vi "MENU7.vi"   [LabVIEW 2015, in "Lazyboots Menu Tool Launch.lvlib"]
uses:
  _Library/Lazyboots Menu Tool Launch.lvlib
  <vilib>/Utility/config.llb/Read Key (String).vi
  <vilib>/Utility/config.llb/NI_LVConfig.lvlib
panel:
  # "Launching..."
types:
  T1 = enum32{"Invalid", "Standard", "Closed", "Hidden", "Minimized", "Maximized"}
  T2 = typedef "NI_LVConfig.lvlib/Config Data RefNum.ctl" = refnum<k1>
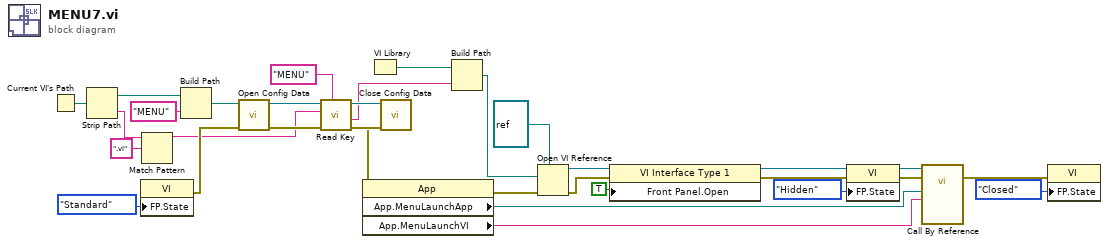
[diagram p0: block diagram]
diagram:
  n1 = Current VI's Path() -> (path=w30:path)
  n2 = Strip Path(path=w30) -> (stripped path=w29:path, name=w19:string)
  n3 = property class="VI"("FP.State"=T1."Standard" ("Front Panel Window:State")) -> (error out=w21:errorcluster)  [unwired: 2 in, 1 out]
  n4 = Match Pattern(string=w19, regular expression=".vi") -> (before substring=w18:string)  [unwired: 4 out]
  n5 = Build Path(base path=w29, name or relative path="MENU") -> (appended path=w27:path)
  n6 = call <vilib>:"Open Config Data.vi"("error in (no error)"=w21, "configuration file path"=w27) -> ("error out"=w25:errorcluster, "refnum"=w26:T2)  [unwired: 7 in, 1 out]
  n7 = call-poly <vilib>:"Read Key.vi"("section"="MENU", "error in (no error)"=w25, "key"=w18, "refnum"=w26) -> ("error out"=w22:errorcluster, "value"=w15:string, "refnum out"=w23:T2)  [unwired: 2 in, 3 out]
  n8 = VI Library() -> (path=w1:path)
  n9 = call <vilib>:"Close Config Data.vi"("error in (no error)"=w22, "refnum"=w23) -> ("error out"=w20:errorcluster)  [unwired: 1 in, 8 out]
  n10 = property class="App"(error in=w20) -> (error out=w14:errorcluster, "App.MenuLaunchApp"=w10:refnum<vi>, "App.MenuLaunchVI"=w9:string)  [unwired: 1 in, 1 out]
  n11 = Build Path(base path=w1, name or relative path=w15) -> (appended path=w16:path)
  n12 = Open VI Reference(type specifier VI Refnum (for type only)=refnum<vi> refnum, vi path=w16, error in (no error)=w14) -> (vi reference=w11:refnum<vi>, error out=w3:errorcluster)  [unwired: 3 out]
  n13 = property class="VI Interface Type 1"(reference=w11, error in=w3, "Front Panel.Open"=TRUE ("Front Panel Window:Open")) -> (reference out=w7:refnum<vi>, error out=w2:errorcluster)
  n14 = property class="VI"(error in=w2, "FP.State"=T1."Hidden" ("Front Panel Window:State")) -> (error out=w4:errorcluster)  [unwired: 1 in, 1 out]
  n15 = call-by-ref "?"(reference=w7, error in=w4, "VI Path"=w9, "Application Reference"=w10) -> (error out=w8:errorcluster)  [unwired: 9 in, 2 out]
  n16 = property class="VI"(error in=w8, "FP.State"=T1."Closed" ("Front Panel Window:State")) -> ()  [unwired: 1 in, 2 out]
